vi "inverz inga.vi"() -> ()   [LabVIEW 2015]
doc: "This VI demonstrates how to control and simulate an inverted pendulum. If you installed the LabVIEW Control Design and Simulation Module, you can design a controller by specifying the pole locations. Otherwise, you can specify the feedback gain matrix."
uses:
  <vilib>/Simulation/Scripting/Companion Diagram/SimConfigNode/SimDog.xnode
  Inverted Pendulum/subVIs/Draw Linear Inverted Pendulum_sim.vi
  <vilib>/addons/Control Design/_State Feedback Control/NI_CD_State Feedback Control.lvlib
  <vilib>/addons/Control Design/_Model Construction/NI_LinSys_Model Creation.lvlib
  <vilib>/addons/Control Design/_Model Construction/Model Creation.llb/Model Creation SubVI/cd_Create State Space Model.vi
  <vilib>/Simulation/Implementation/Shared/SIMSCR Execution Mode.ctl
  <vilib>/Simulation/Scripting/Companion Diagram/SimConfigNode/_simSolvers.ctl
  <vilib>/Simulation/Scripting/Companion Diagram/SimConfigNode/SimParams.ctl
  <vilib>/Simulation/Implementation/XNodeFramework/SimXNode/SimX.xnode
  <vilib>/addons/Control Design/_Utility/NI_CD_Model Viewer.lvlib
  <vilib>/addons/Control Design/_Utility/Model Viewer.llb/Model Viewer SubVI/cd_Draw State-Space Equation (SS).vi
  <vilib>/addons/Control Design/_Dynamic Analysis/NI_CD_Dynamic Analysis.lvlib
  <vilib>/addons/Control Design/_Dynamic Analysis/Dynamic Analysis.llb/Dynamic Analysis subVI/cd_Poles (State-Space).vi
  <vilib>/Simulation/SignalDisplay/Implementation/NILVSim Time Waveform.llb/SIM Time Waveform (vector).vi
  <vilib>/addons/Control Design/_Model Conversions/Simulation Model.llb/CD Convert Simulation to Control Design.vi
  <vilib>/addons/Control Design/_Model Conversions/NI_LinSys_Simulation Model.lvlib
  <vilib>/addons/Control Design/_Model Conversions/Simulation Model.llb/Simulation Model SubVI/CD Convert SIM MIMO State Space to SS.vi
  <vilib>/Simulation/DiscreteLinear/Implementation/NILVSim Discrete State Space Buffered.llb/SIM Discrete State Space Buffered (MIMO).vi
  <vilib>/Simulation/Utility/Implementation/SIM Halt.vi
  <vilib>/Simulation/SignalArithmetic/Implementation/NILVSim Gain.llb/SIM Gain (dot product).vi
  <vilib>/addons/Fuzzy Logic/FL Load Fuzzy System.vi
  <vilib>/addons/Fuzzy Logic/NI_Fuzzy_Logic_API.lvlib
  <vilib>/addons/Control Design/_Model Construction/Model Typedefs.llb/CD General Elements.ctl
  <vilib>/addons/Control Design/_Model Construction/NI_LinSys_Model Typedefs.lvlib
  <vilib>/addons/Control Design/_Model Construction/Model Typedefs.llb/CD State Space Model (MIMO).ctl
panel:
  in  "Disturbance":dbl(slide)=8.99954845277352 scale=-100.0..100.0
  in  "Regulator off?":bool=TRUE
  out "Actual Poles":cdb[](array[numeric]) format="%.2f"
  in  "Feedback Gain":dbl[](array[numeric])=[-168.36531967948676, -87.08873750117637, 222.70457028739702, 44.69540040141787]
  out "State Space Model":picture
  out "3D Picture Control":refnum<vi>(3d-picture)
  out "State-Space Model":T1 {"Transport Delay" format="%.2f"; "D" format="%#.2g"; "C" format="%#.2g"; "B" format="%#.2g"; "A" format="%#.2g"; "properties"."Sampling Time" format="%#.6p"; "properties"."Output Delays" format="%.4f"; "properties"."Input Delays" format="%.4f"}
  in  "Tab":enum32{"Vezérlés tervezés", "Szimuláció"}(tab)
  out "Pole-Zero Map 2":cdb[](graph) caption="Closed-Loop"
  out "Calculated Poles":cdb[](array[numeric])=[-19.999999999997662+0.0i, -15.000000000017264+0.0i, -4.999999999995586+4.2610378298679e-06i, -4.999999999995586-4.2610378298679e-06i] format="%#.2g"
  in  "Desired Poles":cdb[](array[numeric])=[-5.0+0.0i, -5.0+0.0i, -20.0+0.0i, -15.0+0.0i] format="%#.2g"
  out "System Poles":cdb[](array[numeric])=[5.56510798020132+0.0i, -5.60409024766489+0.0i, -0.1428177325364319+0.0i, 0.0+0.0i] format="%#.2g"
  out "Pole-Zero Map":cdb[](graph) caption="Open Loop"
  out "Graph":waveform(dbl)[](graph)=[{"t0"=timestamp(4.71 s since 1904-01-01), "dt"=1.0, "Y"=[-0.13996665083491025]}, {"t0"=timestamp(4.71 s since 1904-01-01), "dt"=1.0, "Y"=[-1.62298383744272e-05]}]
  in  "Setpoint (m)":dbl(slide)=-0.14 scale=-0.2..0.2
  out "Hiba":bool
  out "Measurements (X, Theta)":dbl[](array[numeric])=[-0.13996665083491025, -1.62298383744272e-05] format="%#.4f"
  in  "Stop":bool
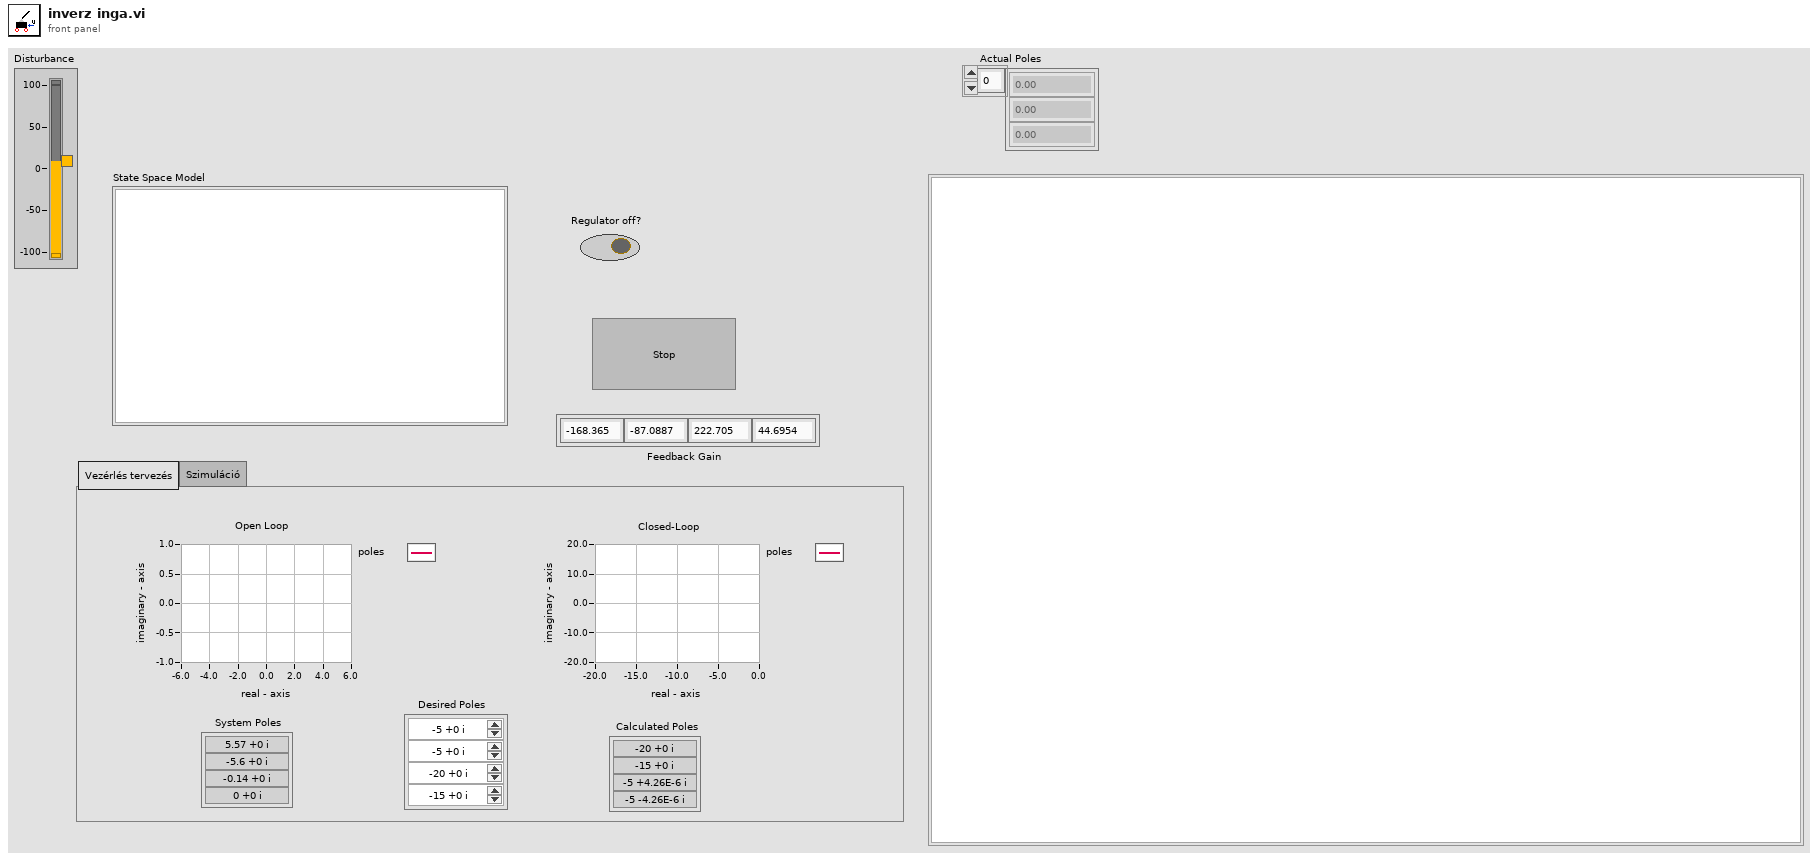
[diagram p1: front panel]
types:
  T1 = typedef "NI_LinSys_Model Typedefs.lvlib/CD State Space Model (MIMO).ctl" = cluster{"properties":T2, "A":dbl[][], "B":dbl[][], "C":dbl[][], "D":dbl[][], "StateNames":string[], "Transport Delay":dbl[][]}
  T2 = typedef "NI_LinSys_Model Typedefs.lvlib/CD General Elements.ctl" = cluster{"Model name":string, "Input names":string[], "Output names":string[], "Input Delays":dbl[], "Output Delays":dbl[], "Sampling Time":dbl, "Notes":string}
  T3 = cluster{"A":dbl[][], "B":dbl[][], "C":dbl[][], "D":dbl[][]}
  T4 = typedef "SimParams.ctl" = cluster{"Initial Time (s)":dbl, "Final Time (s)":dbl, "Step Size (s)":dbl, "ODE Solver":T5, "Minimum Step Size (s)":dbl, "Maximum Step Size (s)":dbl, "Relative Tolerance":dbl, "Absolute Tolerance":dbl, "Software Timing":bool, "Initial Step Size (s)":dbl, "Automatic Fixed Step Size?":bool, "Automatic Discrete Step Size?":bool, "Discrete Step Size (s)":dbl, "Calculate using Time Step":bool, "Solver Wired?":bool, "Prev.Frm.Expected End":u64, "Prev.Frm.Actual End":u64, "Prev.Frm.Finished Late?":bool, "Prev.Iter.Expected End":u64, "Prev.Iter.Actual End":u64, "Prev.Iter.Finished Late?":bool, "Expected Iteration Start":u64, "Actual Iteration Start":u64, "Expected Frame Start":u64, "Actual Frame Start":u64, "Source Name":string, "Name":string, "Period":i64, "Deadline":i64, "Offset":i64, "Start":i64, "Priority":i32, "Timeout":i32, "Processor":i32, "Mode":enum32{"No Change", "Process missed periods, maintain original phase", "Discard missed periods, maintain original phase", "Process missed periods, ignore original phase", "Discard missed periods, ignore original phase"}, "Wakeup reason":enum32{"Normal", "Aborted", "Asynchronous wakeup", "Timing source error", "Timed loop error", "Timeout"}, "Error":errorcluster, "Source Type":string, "Secondary Source Type":string, "Global End Time":u64, "Global Start Time":u64, "Full Solver Reset":bool, "Execution Mode":T6, "Nan/Inf Check":bool, "Custom Solver Library":string, "Solver Is Variable":bool, "custom solver name":string, "Signal Collection Decimation":u32}
  T5 = typedef "_simSolvers.ctl" = enum16{"Runge-Kutta 1 (Euler)", "Runge-Kutta 2", "Runge-Kutta 3", "Runge-Kutta 4", "Runge-Kutta 23 (variable)", "Runge-Kutta 45 (variable)", "BDF (variable)", "Adams-Moulton (variable)", "Rosenbrock (variable)", "Discrete States Only", "SDIRK 4 (variable)", "Radau 5 (variable)", "Radau 9 (variable)", "Radau 13 (variable)", "Radau [Variable Order] (variable)", "Gear's Method (variable)", "Linearizer", "State Query", "Trim Eval", "Custom Solver"}
  T6 = typedef "SIMSCR Execution Mode.ctl" = enum16{"Simulate to Completion", "Single Time-Step Simulation (Fixed Step Only)"}
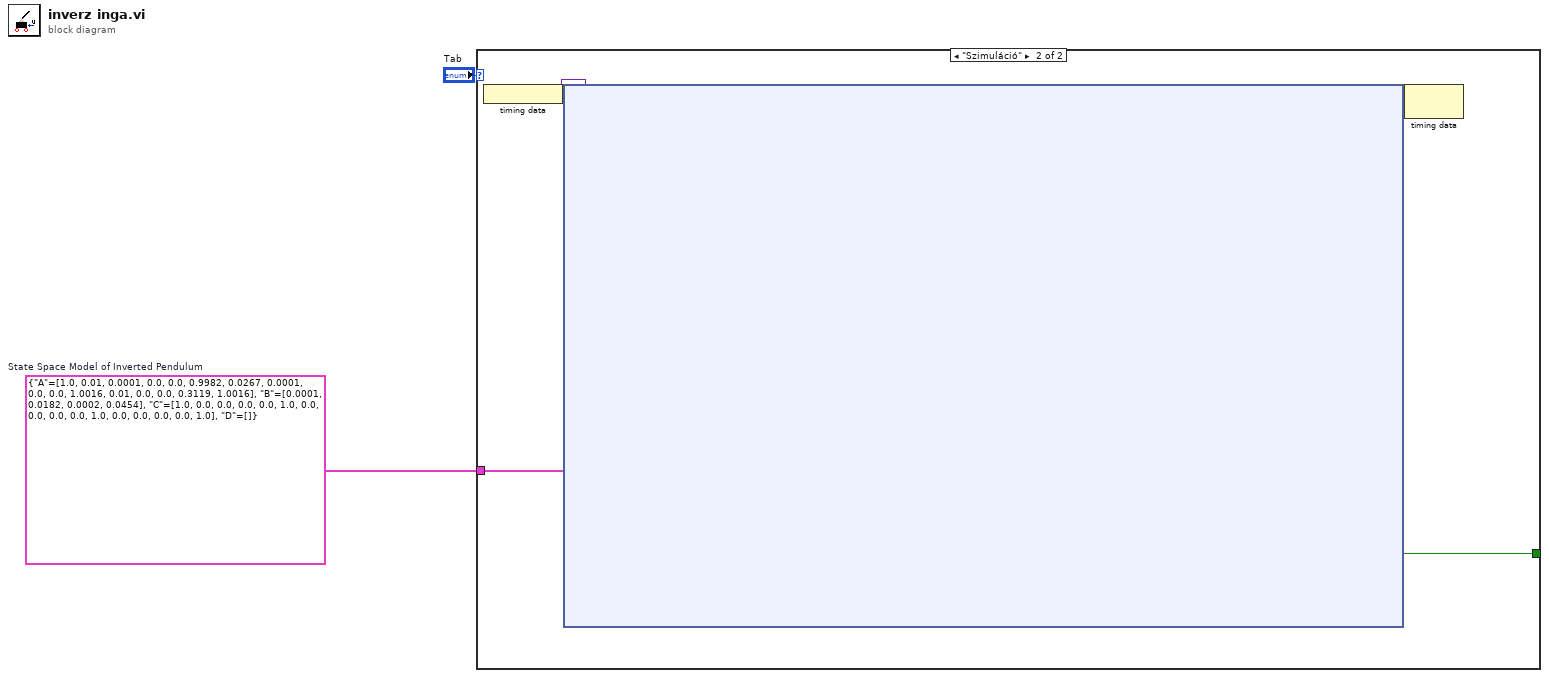
[diagram p0: block diagram]
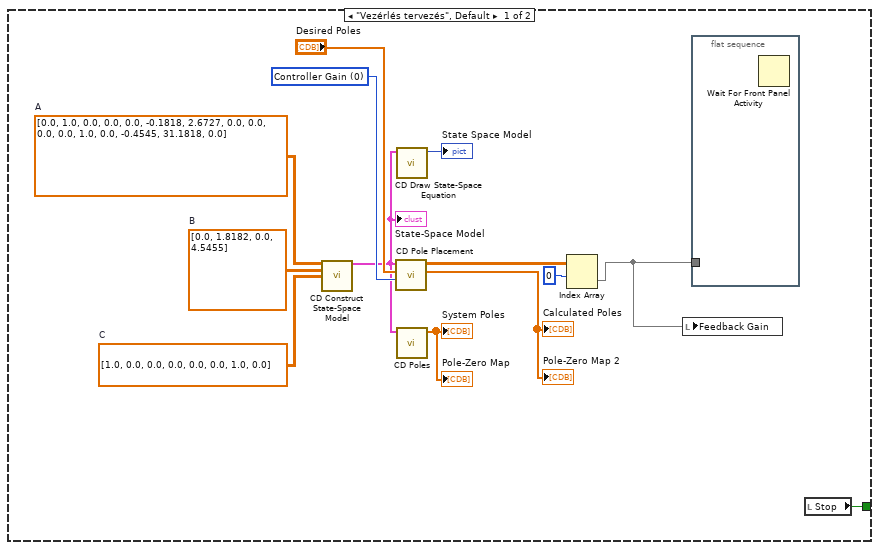
[diagram p2: hidden frame]
diagram:
  w2 = T3 {"A"=[[1.0, 0.01, 0.0001, 0.0], [0.0, 0.9982, 0.0267, 0.0001], [0.0, 0.0, 1.0016, 0.01], [0.0, 0.0, 0.3119, 1.0016]], "B"=[[0.0001], [0.0182], [0.0002], [0.0454]], "C"=[[1.0, 0.0, 0.0, 0.0], [0.0, 1.0, 0.0, 0.0], [0.0, 0.0, 1.0, 0.0], [0.0, 0.0, 0.0, 1.0]], "D"=[]}  # State Space Model of Inverted Pendulum
  n1 = case shown="\"Szimuláció\"" "Tab" {
    tunnel: [w8 w17] -> _
    tunnel: w2 -> [_ w16]
    frame "Vezérlés tervezés", Default {
      w15 = dbl[][] [[1.0, 0.0, 0.0, 0.0], [0.0, 0.0, 1.0, 0.0]]  # C
      w14 = dbl[][] [[0.0], [1.8182], [0.0], [4.5455]]  # B
      w13 = dbl[][] [[0.0, 1.0, 0.0, 0.0], [0.0, -0.1818, 2.6727, 0.0], [0.0, 0.0, 0.0, 1.0], [0.0, -0.4545, 31.1818, 0.0]]  # A
      w9 = u16 0 items=["Controller Gain", "Observer Gain (Predictive)", "Observer Gain (Current)"] ("Gain Type")
      n2 = call-poly <vilib>:"CD Construct State-Space Model.vi"("A"=w13, "B"=w14, "C"=w15) -> ("State-Space Model"=w6:T1)  [unwired: 11 in, 1 out]
      "State-Space Model" <- w6
      n3 = call <vilib>:"CD Pole Placement.vi"("Gain Type"=w9, "Poles"="Desired Poles", "State-Space Model"=w6) -> ("Actual Poles"=→"Calculated Poles" →"Pole-Zero Map 2":cdb[], "Gain"=w11:dbl[][])  [unwired: 6 in, 1 out]
      n4 = call-poly <vilib>:"CD Draw State-Space Equation.vi"("State-Space Model"=w6) -> ("Equation"=→"State Space Model":picture)  [unwired: 8 in, 2 out]
      n5 = call-poly <vilib>:"CD Poles.vi"("State-Space Model"=w6) -> ("Poles"=→"System Poles" →"Pole-Zero Map":cdb[])  [unwired: 9 in, 1 out]
      n6 = Index Array(array=w11, index (row)=0) -> (element=w3:dbl[])  [unwired: 1 in]
      n7 = local write "Feedback Gain"(w3) -> ()
      n8 = flat-sequence {
        tunnel: w3 -> [_]
        frame #0 {
          n9 = Wait For Front Panel Activity() -> ()  [unwired: 3 in, 1 out]
        }
      }
      n10 = local read "Stop"() -> (w8:bool)
    }
    frame "Szimuláció" {
      n11 = node-c288() -> (w19:variant)
      n12 = node-c254 ("Simulation Loop")(w19, w16) -> (w18:variant, w17:bool)
      n13 = node-c288(w18) -> ()  [unwired: 1 out]
    }
  }
